vi "poly_recursive_set_cluster_element(m).vi"(6 "stop after 1st? (T)":bool=TRUE, 7 "delimiter (/)":string="/", 8 "error in (no error)":errorcluster, 9 "field names":string[](array[string]), 10 "data":variant[](array[variant]), 11 "Cluster":variant) -> (0 "error out":errorcluster, 2 "set?":bool[](array[boolean]), 3 "Cluster out":variant)   [LabVIEW 2015]
uses:
  <vilib>/Utility/Data Type/NI_Data Type.lvlib
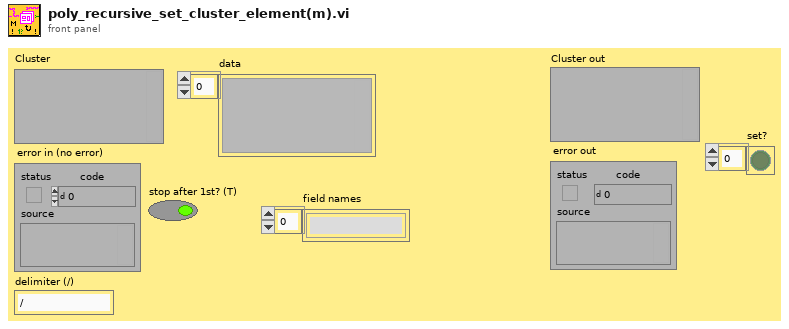
[diagram p1: front panel]
types:
  T1 = typedef "NI_Data Type.lvlib/Data Type.ctl" = enum8{"Invalid Type", "Void", "I8", "I16", "I32", "I64", "U8", "U16", "U32", "U64", "Single Float", "Double Float", "Extended Float", "Single Complex", "Double Complex", "Extended Complex", "Enum U8", "Enum U16", "Enum U32", "Enum U64", "Single Float With Unit", "Double Float With Unit", "Extended Float With Unit", "Single Complex with Unit", "Double Complex with Unit", "Extended Complex with Unit", "Boolean", "String", "Path", "Picture", "Tag", "Array", "Cluster", "Variant", "LV Variant", "Waveform", "Timestamp", "Digital Waveform", "Digital Data", "ExpressData", "Refnum", "External Data", "VI", "Poly VI", "LabVIEW Class Instance", "Fixed Point"}
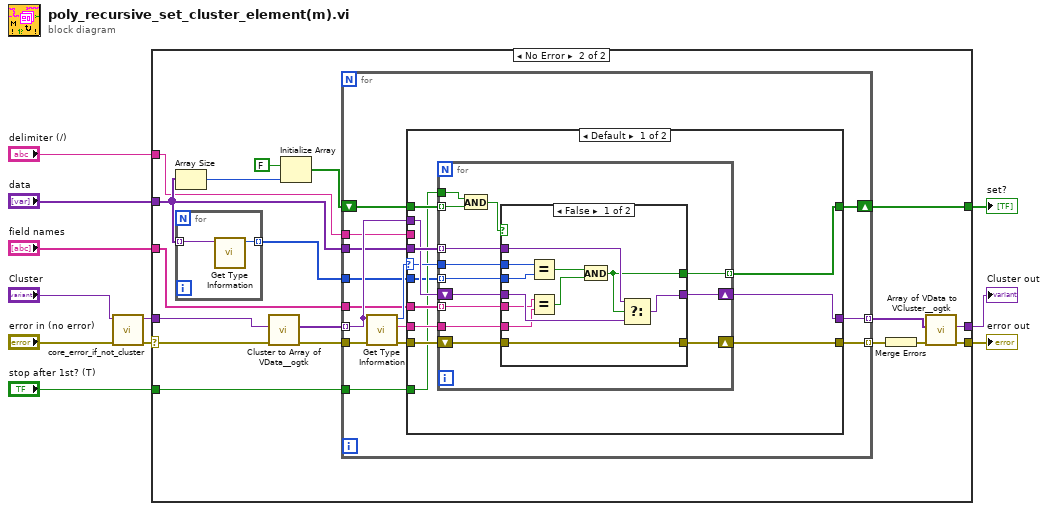
[diagram p0: block diagram]
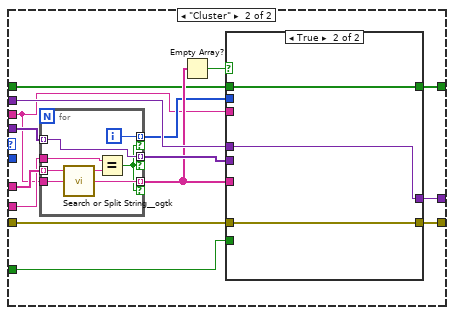
[diagram p4: hidden frame]
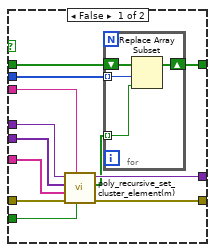
[diagram p5: hidden frame]
diagram:
  n1 = call "core_error_if_not_cluster.vi"("Error in"="error in (no error)", "Cluster"="Cluster") -> ("Error out"=w2:errorcluster, "Cluster duplicate"=w3:variant)  [unwired: 8 in]
  n2 = case shown="No Error" w2 {
    selector: w2 -> [w12 w14]
    tunnel: w3 -> [_ w29]
    tunnel: [_ w26] -> w11
    tunnel: "data" -> [_ w16]
    tunnel: [w12 w23] -> w10
    tunnel: "field names" -> [_ w22]
    tunnel: "stop after 1st? (T)" -> [_ w21]
    tunnel: [_ w18] -> w6
    tunnel: "delimiter (/)" -> [_ w13]
    frame Error {
    }
    frame No Error {
      n3 = Array Size(array=w16) -> (size(s)=w19:i32)
      n4 = for {
        tunnel: w16 -> [w32] mode=indexing
        tunnel: [w31] -> w15 mode=indexing
        n5 = call <vilib>:"Get Type Information.vi"("Variant"=w32) -> ("Type"=w31:T1)  [unwired: 6 in, 4 out]
      }
      n6 = call <userlib>:"Cluster to Array of VData__ogtk.vi"("error in (no error)"=w14, "Cluster"=w29) -> ("error out"=w28:errorcluster, "Array of VData"=w30:variant[])  [unwired: 8 in]
      n7 = Initialize Array ("element has been replaced")(FALSE, w19) -> (w17:bool[])
      n8 = for {
        tunnel: w30 -> [w45] mode=indexing
        tunnel: [w46] -> w27 mode=indexing
        tunnel: w16 -> [w43]
        tunnel: [w40] -> w25 mode=indexing
        tunnel: w28 -> [w42]
        tunnel: w22 -> [w39]
        tunnel: w21 -> [w37]
        shift-right: [w36] -> w18
        shift-left: w17 -> [w35]
        tunnel: w15 -> [w34]
        tunnel: w13 -> [w33]
        n9 = call <vilib>:"Get Type Information.vi"("error in (no error)"=w42, "Variant"=w45) -> ("error out"=w41:errorcluster, "Name"=w38:string, "Type"=w44:T1)  [unwired: 5 in, 2 out]
        n10 = case shown="Default" w44 {
          selector: w44 -> [w52 _]
          tunnel: [w58 w97] -> w46
          tunnel: w45 -> [w54 w98]
          tunnel: w43 -> [w55 w93]
          tunnel: w41 -> [w57 w100]
          tunnel: [w56 w99] -> w40
          tunnel: w39 -> [w53 w96]
          tunnel: w38 -> [w51 w95]
          tunnel: w35 -> [w50 w89]
          tunnel: [w49 w90] -> w36
          tunnel: w37 -> [w48 w87]
          tunnel: w34 -> [w47 _]
          tunnel: w33 -> [_ w86]
          frame Default {
            n11 = for {
              tunnel: w55 -> [w69] mode=indexing
              tunnel: w53 -> [w67] mode=indexing
              shift-right: [w70] -> w56
              shift-left: w57 -> [w64]
              shift-right: [w71] -> w58
              shift-left: w54 -> [w68]
              tunnel: w52 -> [w66]
              tunnel: w51 -> [w65]
              tunnel: [w63] -> w49 mode=indexing
              tunnel: w50 -> [w62] mode=indexing
              tunnel: w48 -> [w60]
              tunnel: w47 -> [w59] mode=indexing
              n12 = And(x=w60, y=w62) -> (x .and. y?=w61:bool)
              n13 = case shown="False" w61 {
                selector: w61 -> [_ w85]
                tunnel: [w82 w84] -> w71
                tunnel: [w72 w83] -> w70
                tunnel: w69 -> [w79 _]
                tunnel: w68 -> [w78 w84]
                tunnel: w67 -> [w77 _]
                tunnel: w66 -> [w76 _]
                tunnel: w65 -> [w75 _]
                tunnel: w64 -> [w72 w83]
                tunnel: [w74 w85] -> w63
                tunnel: w59 -> [w73 _]
                frame False {
                  n14 = Equal?(x=w76, y=w73) -> (x = y?=w81:bool)
                  n15 = Equal?(x=w77, y=w75) -> (x = y?=w80:bool)
                  n16 = And(x=w81, y=w80) -> (x .and. y?=w74:bool)
                  n17 = Select(t=w79, s=w74, f=w78) -> (s? t:f=w82:variant)
                }
                frame True {
                }
              }
            }
          }
          frame "Cluster" {
            n18 = for {
              tunnel: w96 -> [w108] mode=indexing
              tunnel: [w107] -> w92 mode=indexing if=w102
              tunnel: w95 -> [w106]
              tunnel: [w104] -> w94 mode=indexing if=w102
              tunnel: w93 -> [w104] mode=indexing
              tunnel: [w103] -> w88 mode=indexing if=w102
              tunnel: w86 -> [w101]
              i -> [w103]
              n19 = call <userlib>:"Search or Split String__ogtk.vi"("search string/char (-)"=w101, "string"=w108) -> ("substring after match"=w107:string, "substring before match"=w105:string)  [unwired: 1 in, 1 out]
              n20 = Equal?(x=w106, y=w105) -> (x = y?=w102:bool)
            }
            n21 = Empty Array?(array=w92) -> (empty?=w91:bool)
            n22 = case shown="True" w91 {
              tunnel: w100 -> [w120 w126]
              tunnel: [w119 w126] -> w99
              tunnel: w98 -> [w118 w127]
              tunnel: w94 -> [w117 _]
              tunnel: [w116 w127] -> w97
              tunnel: w92 -> [w115 _]
              tunnel: [w111 w125] -> w90
              tunnel: w89 -> [w112 w125]
              tunnel: w88 -> [w114 _]
              tunnel: w87 -> [w110 _]
              tunnel: w86 -> [w109 _]
              frame False {
                n23 = call "poly_recursive_set_cluster_element(m).vi"("stop after 1st? (T)"=w110, "delimiter (/)"=w109, "error in (no error)"=w120, "field names"=w115, "data"=w117, "Cluster"=w118) -> ("error out"=w119:errorcluster, "set?"=w113:bool[], "Cluster out"=w116:variant)  [unwired: 3 in]
                n24 = for {
                  tunnel: w114 -> [w124] mode=indexing
                  tunnel: w113 -> [w123] mode=indexing
                  shift-right: [w121] -> w111
                  shift-left: w112 -> [w122]
                  n25 = Replace Array Subset(array=w122, new element=w123, index=w124) -> (w121:bool[])
                }
              }
              frame True {
              }
            }
          }
        }
      }
      n26 = Merge Errors(w25) -> (w24:errorcluster)
      n27 = call <userlib>:"Array of VData to VCluster__ogtk.vi"("error in (no error)"=w24, "Array"=w27) -> ("error out"=w23:errorcluster, "VCluster"=w26:variant)  [unwired: 8 in]
    }
  }
  "Cluster out" <- w11
  "error out" <- w10
  "set?" <- w6
